vi "otsu.vi"() -> ()   [LabVIEW 2026]
uses:
  <vilib>/vision/NI_Vision_Development_Module.lvlib
panel:
  out "Threshold Range Out":cluster{"Lower value":sgl, "Upper value":sgl}={"Lower value"=128.0, "Upper value"=255.0} {"Upper value" format="%.2f"; "Lower value" format="%.2f"}
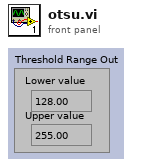
[diagram p1: front panel]
types:
  T1 = typedef "Image Type" = u32
  T2 = typedef "IMAQ Image.ctl" = refnum<image>
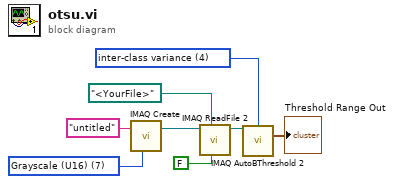
[diagram p0: block diagram]
diagram:
  w2 = 4 items=["clustering", "entropy", "metric", "moments", "inter-class variance"] ("Method (clustering)")
  w4 = T1 7 items=["Grayscale (U8)", "Grayscale (I16)", "Grayscale (SGL)", "Complex (CSG)", "RGB (U32)", "HSL (U32)", "RGB (U64)", "Grayscale (U16)"] ("Image Type")
  n1 = call "IMAQ Create"("Image Name"="untitled", "Image Type"=w4) -> ("New Image"=w7:T2)  [unwired: 3 in, 1 out]
  n2 = call "IMAQ ReadFile 2"("Use File Path Image Type"=FALSE, "File Path"=path "<YourFile>", "Image"=w7) -> ("Image Out"=w3:T2)  [unwired: 4 in, 4 out]
  n3 = call "IMAQ AutoBThreshold 2"("Image Src"=w3, "Method (clustering)"=w2) -> ("Threshold Range Out"=→"Threshold Range Out":cluster{"Lower value":sgl, "Upper value":sgl})  [unwired: 11 in, 2 out]
